vi "Latch on Falling.vi"(5 "Boolean in":bool) -> (2 "Boolean out":bool)   [LabVIEW 2016]
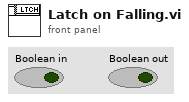
[diagram p1: front panel]
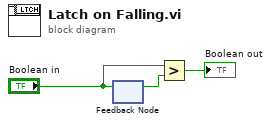
[diagram p0: block diagram]
diagram:
  n1 = feedback #1() -> (w2:bool)  [unwired: 1 in]
  n2 = feedback-in #1("Boolean in") -> ()
  n3 = Greater?(x="Boolean in", y=w2) -> (0:→"Boolean out":bool)
